vi "Save data file to network drive v1.vi"(11 "panel id":string) -> (0 "network file save error":errorcluster, 3 "file save path":string)   [LabVIEW 2013]
uses:
  program files/Global 1.vi
  program files/Global display 2.vi
  program files/Global display 3.vi
panel:
  out "C drive root path":string
  out "network file dir path":path
  out "network dir":string
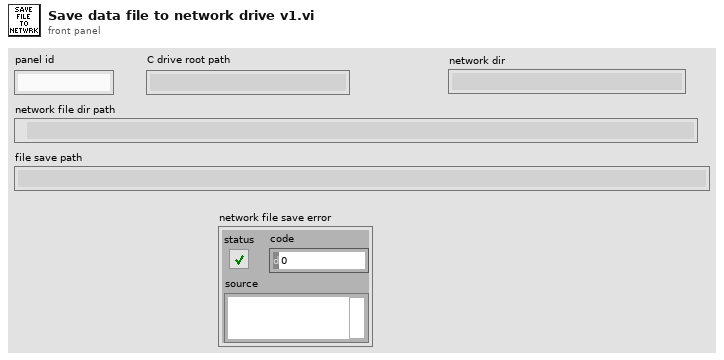
[diagram p1: front panel]
types:
  T1 = cluster{"CYCLE":dbl, "MINS":dbl, "STATUS":string}
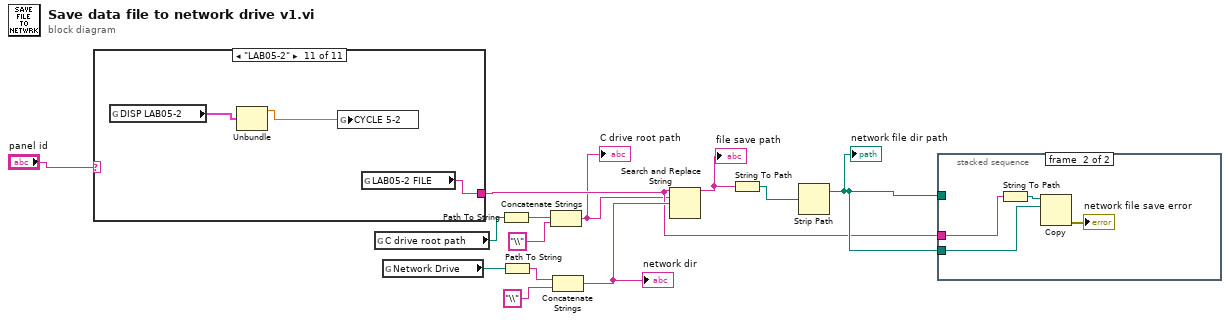
[diagram p0: block diagram]
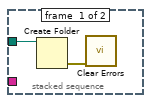
[diagram p2: hidden frame]
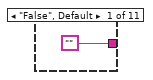
[diagram p3: hidden frame]
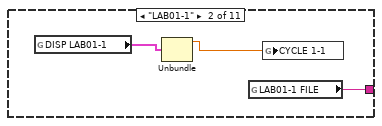
[diagram p4: hidden frame]
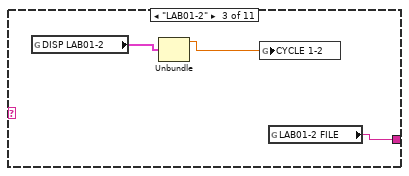
[diagram p5: hidden frame]
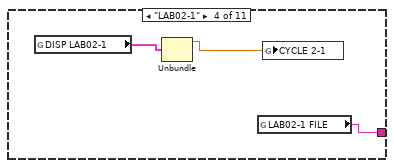
[diagram p6: hidden frame]
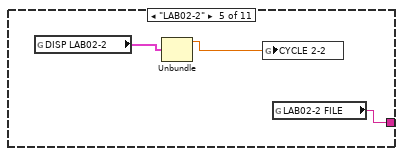
[diagram p7: hidden frame]
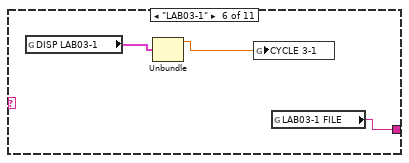
[diagram p8: hidden frame]
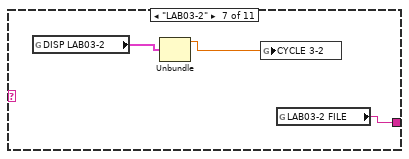
[diagram p9: hidden frame]
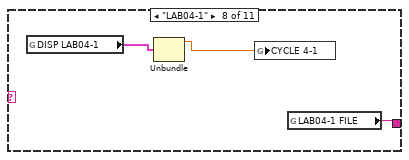
[diagram p10: hidden frame]
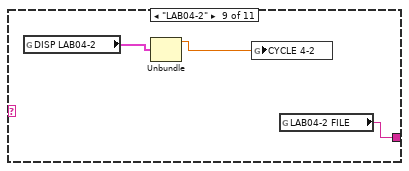
[diagram p11: hidden frame]
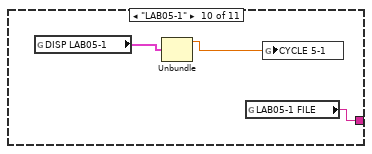
[diagram p12: hidden frame]
diagram:
  n1 = case shown="\"LAB05-2\"" "panel id" {
    tunnel: ["" w17 w20 w23 w26 w29 w32 w35 w38 w41 w44] -> w5
    frame "False", Default {
    }
    frame "LAB01-1" {
      n2 = global read "Global display 2.vi" "DISP LAB01-1"() -> (w16:T1)
      n3 = Unbundle(w16) -> ("CYCLE"=w15:dbl)  [unwired: 2 out]
      n4 = global read "Global 1.vi" "LAB01-1 FILE"() -> (w17:string)
      n5 = global write "Global display 3.vi" "CYCLE 1-1"(w15) -> ()
    }
    frame "LAB01-2" {
      n6 = global read "Global display 2.vi" "DISP LAB01-2"() -> (w19:T1)
      n7 = Unbundle(w19) -> ("CYCLE"=w18:dbl)  [unwired: 2 out]
      n8 = global write "Global display 3.vi" "CYCLE 1-2"(w18) -> ()
      n9 = global read "Global 1.vi" "LAB01-2 FILE"() -> (w20:string)
    }
    frame "LAB02-1" {
      n10 = global read "Global display 2.vi" "DISP LAB02-1"() -> (w22:T1)
      n11 = Unbundle(w22) -> ("CYCLE"=w21:dbl)  [unwired: 2 out]
      n12 = global read "Global 1.vi" "LAB02-1 FILE"() -> (w23:string)
      n13 = global write "Global display 3.vi" "CYCLE 2-1"(w21) -> ()
    }
    frame "LAB02-2" {
      n14 = global read "Global display 2.vi" "DISP LAB02-2"() -> (w25:T1)
      n15 = Unbundle(w25) -> ("CYCLE"=w24:dbl)  [unwired: 2 out]
      n16 = global write "Global display 3.vi" "CYCLE 2-2"(w24) -> ()
      n17 = global read "Global 1.vi" "LAB02-2 FILE"() -> (w26:string)
    }
    frame "LAB03-1" {
      n18 = global read "Global display 2.vi" "DISP LAB03-1"() -> (w28:T1)
      n19 = Unbundle(w28) -> ("CYCLE"=w27:dbl)  [unwired: 2 out]
      n20 = global write "Global display 3.vi" "CYCLE 3-1"(w27) -> ()
      n21 = global read "Global 1.vi" "LAB03-1 FILE"() -> (w29:string)
    }
    frame "LAB03-2" {
      n22 = global read "Global display 2.vi" "DISP LAB03-2"() -> (w31:T1)
      n23 = Unbundle(w31) -> ("CYCLE"=w30:dbl)  [unwired: 2 out]
      n24 = global write "Global display 3.vi" "CYCLE 3-2"(w30) -> ()
      n25 = global read "Global 1.vi" "LAB03-2 FILE"() -> (w32:string)
    }
    frame "LAB04-1" {
      n26 = global read "Global display 2.vi" "DISP LAB04-1"() -> (w34:T1)
      n27 = Unbundle(w34) -> ("CYCLE"=w33:dbl)  [unwired: 2 out]
      n28 = global write "Global display 3.vi" "CYCLE 4-1"(w33) -> ()
      n29 = global read "Global 1.vi" "LAB04-1 FILE"() -> (w35:string)
    }
    frame "LAB04-2" {
      n30 = global read "Global display 2.vi" "DISP LAB04-2"() -> (w37:T1)
      n31 = Unbundle(w37) -> ("CYCLE"=w36:dbl)  [unwired: 2 out]
      n32 = global write "Global display 3.vi" "CYCLE 4-2"(w36) -> ()
      n33 = global read "Global 1.vi" "LAB04-2 FILE"() -> (w38:string)
    }
    frame "LAB05-1" {
      n34 = global read "Global display 2.vi" "DISP LAB05-1"() -> (w40:T1)
      n35 = Unbundle(w40) -> ("CYCLE"=w39:dbl)  [unwired: 2 out]
      n36 = global read "Global 1.vi" "LAB05-1 FILE"() -> (w41:string)
      n37 = global write "Global display 3.vi" "CYCLE 5-1"(w39) -> ()
    }
    frame "LAB05-2" {
      n38 = global read "Global display 2.vi" "DISP LAB05-2"() -> (w43:T1)
      n39 = Unbundle(w43) -> ("CYCLE"=w42:dbl)  [unwired: 2 out]
      n40 = global write "Global display 3.vi" "CYCLE 5-2"(w42) -> ()
      n41 = global read "Global 1.vi" "LAB05-2 FILE"() -> (w44:string)
    }
  }
  n42 = global read "Global 1.vi" "C drive root path"() -> (w2:path)
  n43 = global read "Global 1.vi" "Network Drive"() -> (w12:path)
  n44 = Path To String(path=w2) -> (string=w3:string)
  n45 = Path To String(path=w12) -> (string=w11:string)
  n46 = Concatenate Strings(w3, "\\") -> (w1:string)
  "C drive root path" <- w1
  n47 = Concatenate Strings(w11, "\\") -> (w9:string)
  "network dir" <- w9
  n48 = Search and Replace String(input string=w5, search string=w1, replace string=w9) -> (result string=w8:string)  [unwired: 5 in, 3 out]
  "file save path" <- w8
  n49 = String To Path(string=w8) -> (path=w7:path)
  n50 = Strip Path(path=w7) -> (stripped path=w6:path)  [unwired: 1 out]
  "network file dir path" <- w6
  n51 = stacked-sequence {
    tunnel: w6 -> [w46 _]
    tunnel: w5 -> [_ w48]
    tunnel: w6 -> [_ w47]
    frame #0 {
      n52 = Create Folder(path (use dialog)=w46) -> (error out=w45:errorcluster)  [unwired: 2 in, 2 out]
      n53 = call <vilib>:"Clear Errors.vi"("error in (no error)"=w45) -> ()  [unwired: 6 in, 1 out]
    }
    frame #1 {
      n54 = String To Path(string=w48) -> (path=w49:path)
      n55 = Copy(10:w47, 11:w49) -> (0:→"network file save error":errorcluster)  [unwired: 3 in, 2 out]
    }
  }
